vi "POST_Method.vi"() -> ()   [LabVIEW 2017]
uses:
  <vilib>/httpClient/POSTBuffer.vi
  <vilib>/httpClient/LabVIEWHTTPClient.lvlib
panel:
  out "body":string
  out "headers":string
  in  "dC":dbl(slide) scale=0.0..300.0
  in  "dB":dbl(slide) scale=0.0..300.0
  in  "dA":dbl(slide) scale=0.0..300.0
  in  "stop":bool
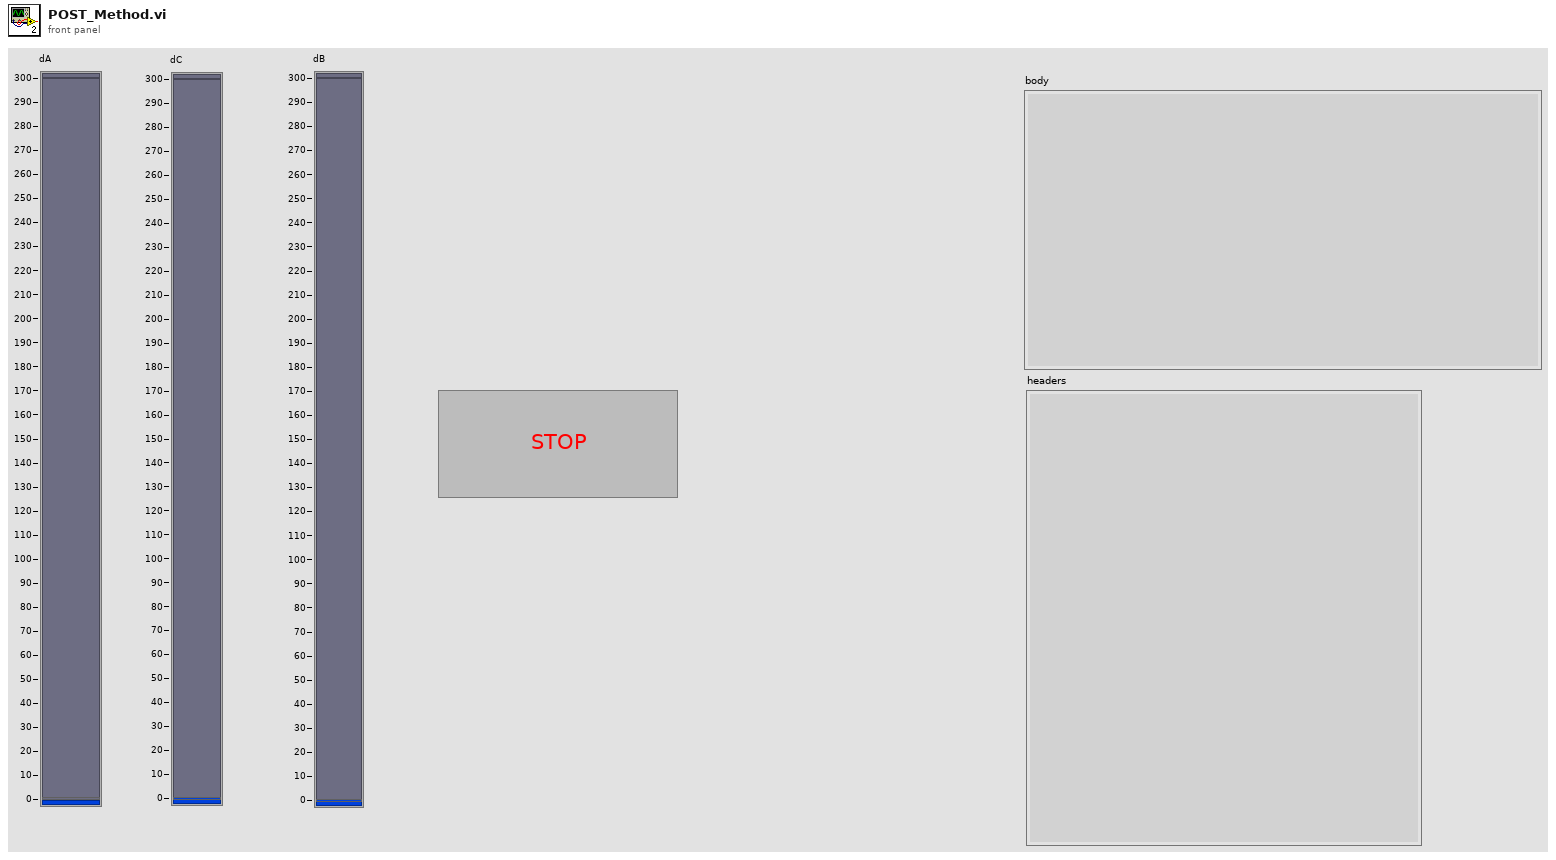
[diagram p1: front panel]
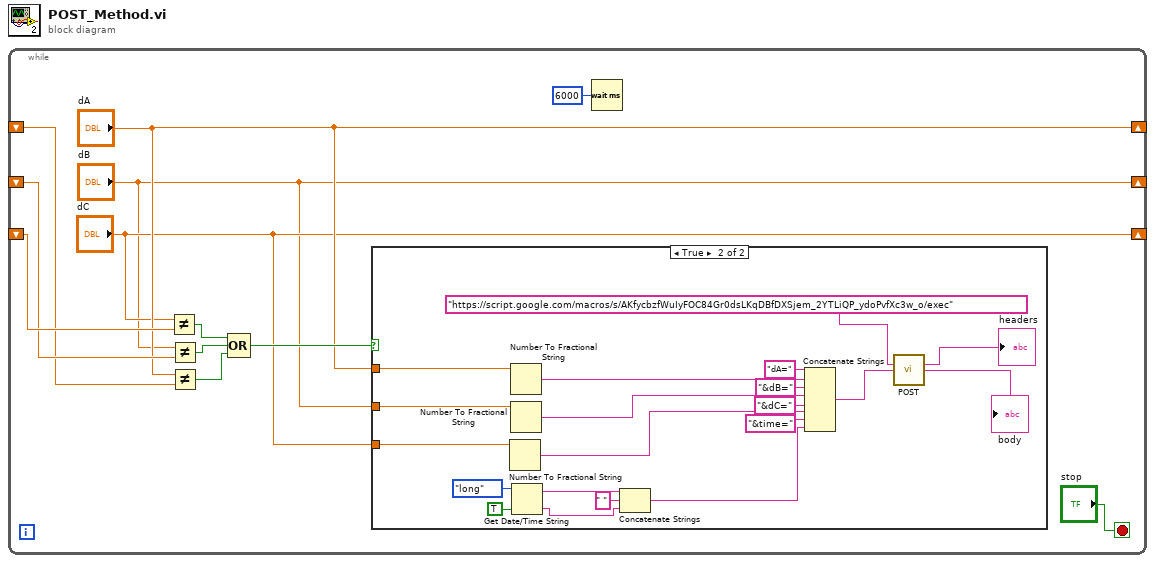
[diagram p0: block diagram]
diagram:
  n1 = while {
    shift-right: ["dC"] -> _
    shift-left: _ -> [w12]
    shift-right: ["dB"] -> _
    shift-left: _ -> [w7]
    shift-right: ["dA"] -> _
    shift-left: _ -> [w6]
    stop <- "stop" stop-if-true
    n2 = Not Equal?(x="dC", y=w12) -> (x != y?=w11:bool)
    n3 = Not Equal?(x="dB", y=w7) -> (x != y?=w10:bool)
    n4 = Not Equal?(x="dA", y=w6) -> (x != y?=w9:bool)
    n5 = Compound Arithmetic op=OR(w11, w10, w9) -> (w8:bool)
    n6 = case shown="True" w8 {
      tunnel: "dC" -> [_ w30]
      tunnel: "dB" -> [_ w31]
      tunnel: "dA" -> [_ w32]
      frame False {
      }
      frame True {
        n7 = Number To Fractional String(number=w30) -> (F-format string=w25:string)  [unwired: 3 in]
        n8 = Number To Fractional String(number=w32) -> (F-format string=w29:string)  [unwired: 3 in]
        n9 = Number To Fractional String(number=w31) -> (F-format string=w27:string)  [unwired: 3 in]
        n10 = Get Date/Time String(date format (0)=enum16{"short", "long", "abbreviated"}."long", want seconds? (F)=TRUE) -> (date string=w21:string, time string=w19:string)  [unwired: 1 in]
        n11 = Concatenate Strings(w21, " " ("string"), w19) -> (w18:string)
        n12 = Concatenate Strings("dA=" ("string"), w29, "&dB=" ("string"), w27, "&dC=" ("string"), w25, "&time=" ("string"), w18) -> (w15:string)
        n13 = call-poly <vilib>:"POST.vi"("url"="https://script.google.com/macros/s/AKfycbzfWuIyFOC84Gr0dsLKqDBfDXSjem_2YTLiQP_ydoPvfXc3w_o/exec", "buffer"=w15) -> ("headers"=→"headers":string, "body"=→"body":string)  [unwired: 10 in, 2 out]
      }
    }
    n14 = Wait (ms)(milliseconds to wait=u32 6000) -> ()  [unwired: 1 out]
  }
